vi "Cleanup Futures.vi"(8 "error in (no error)":errorcluster, 11 "Future in":refnum<class "Future.lvclass">[](array[class])) -> ()   [LabVIEW 2020, in "Promises.lvlib" / "Future.lvclass"]
uses:
  Future.lvclass
  Future.lvclass/Future.ctl
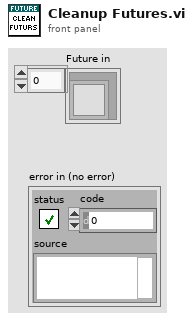
[diagram p1: front panel]
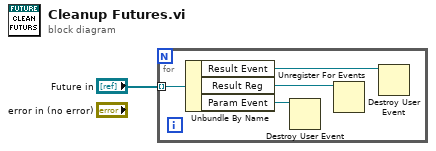
[diagram p0: block diagram]
diagram:
  n1 = for {
    tunnel: "Future in" -> [w5] mode=indexing
    n2 = Unbundle By Name(w5) -> ("Result Event"=w2:refnum<user-event>, "Result Reg"=w3:refnum<event-registration>, "Param Event"=w4:refnum<user-event>)
    n3 = Destroy User Event(user event=w4) -> ()  [unwired: 1 in, 1 out]
    n4 = Unregister For Events(event registration refnum=w3) -> ()  [unwired: 1 in, 1 out]
    n5 = Destroy User Event(user event=w2) -> ()  [unwired: 1 in, 1 out]
  }
